vi "Text for boolean selector.vi"(7 "C1 op C2":T1) -> (8 "String":string)   [LabVIEW 2011]
uses:
  Boolean operation.ctl
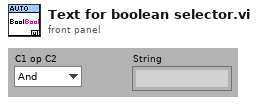
[diagram p1: front panel]
types:
  T1 = typedef "Boolean operation.ctl" = enum16{"And", "Or", "Xor", "Nand", "Nor", "Nxor", "Implies"}
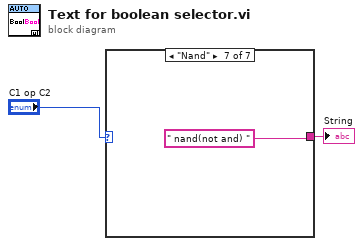
[diagram p0: block diagram]
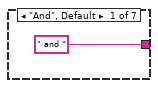
[diagram p2: hidden frame]
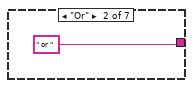
[diagram p3: hidden frame]
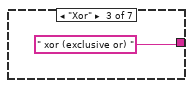
[diagram p4: hidden frame]
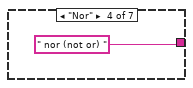
[diagram p5: hidden frame]
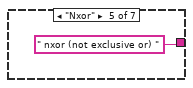
[diagram p6: hidden frame]
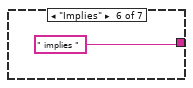
[diagram p7: hidden frame]
diagram:
  n1 = case shown="\"Nand\"" "C1 op C2" {
    tunnel: [" and " " or " " xor (exclusive or) " " nor (not or) " " nxor (not exclusive or) " " implies " " nand(not and) "] -> w2
    frame "And", Default {
    }
    frame "Or" {
    }
    frame "Xor" {
    }
    frame "Nor" {
    }
    frame "Nxor" {
    }
    frame "Implies" {
    }
    frame "Nand" {
    }
  }
  "String" <- w2
